vi "Start Cooker.vi"(8 "error in (no error)":errorcluster, 11 "COOKING in":refnum<class "COOKING.lvclass">) -> (0 "error out":errorcluster, 3 "COOKING out":refnum<class "COOKING.lvclass">)   [LabVIEW 2024, in "Chef States.lvlib" / "COOKING.lvclass"]
uses:
  COOKING.lvclass
  Cooker Actor/Cooker Actor Messages/Start Msg/Start Msg.lvclass/Start Msg.ctl
  <vilib>/ActorFramework/Message Enqueuer/Message Enqueuer.lvclass/Message Enqueuer.ctl
  <vilib>/ActorFramework/Message Enqueuer/Enqueue.vi
  Cooker Actor/Cooker Actor Messages/Start Msg/Start Msg.lvclass
  C:/Program Files/National Instruments/LabVIEW 2024/vi.lib/ActorFramework/Message/Message.lvclass
  <vilib>/ActorFramework/Message Priority Queue/Priority Enqueue.vi
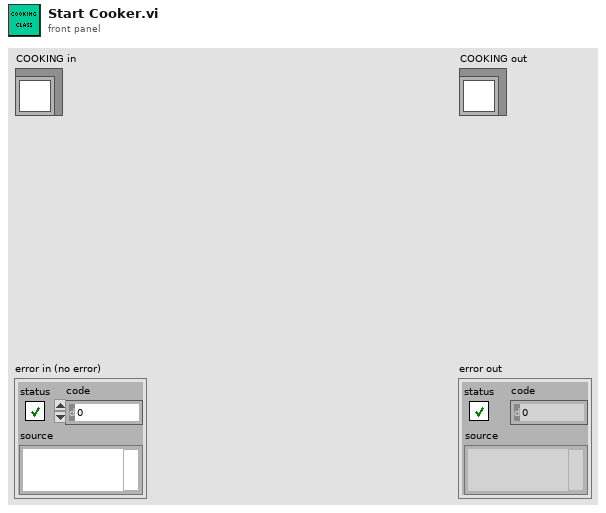
[diagram p1: front panel]
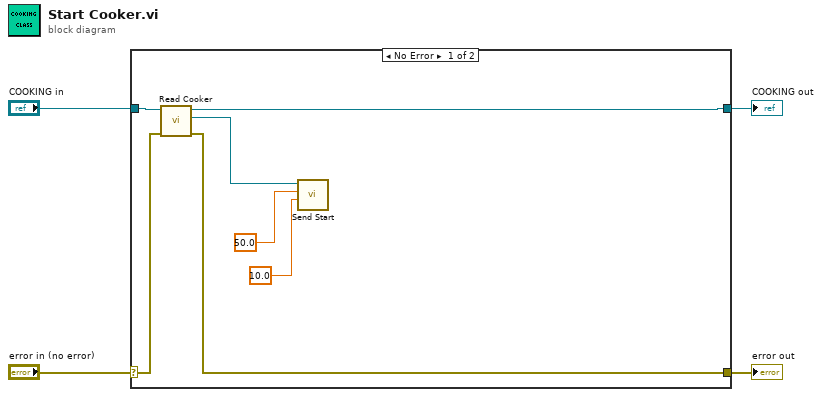
[diagram p0: block diagram]
diagram:
  n1 = case shown="No Error" "error in (no error)" {
    selector: "error in (no error)" -> [w11 w13]
    tunnel: [w10 w13] -> w3
    tunnel: [w8 w12] -> w1
    tunnel: "COOKING in" -> [w9 w12]
    frame No Error {
      n2 = call-dynamic "Read Cooker.vi"("error in (no error)"=w11, "Chef State in"=w9) -> ("error out"=w10:errorcluster, "Actor Framework:Message Enqueuer"=w7:refnum<class "Message Enqueuer.lvclass">, "Chef State out"=w8:refnum<class "COOKING.lvclass">)  [unwired: 7 in]
      n3 = call "Send Start.vi"("Duration (s)"=10.0, "Set Fire (%)"=50.0, "Message Enqueuer"=w7) -> ()  [unwired: 7 in, 2 out]
    }
    frame Error {
    }
  }
  "error out" <- w3
  "COOKING out" <- w1
